vi "Costruisci rampa.vi"(11 "Cluster rampa":T2={"Numero step totali"=10.0, "Tempo step [s]"=1.0, "Freno"={"MARCIA"=FALSE, "Control Type"=enum."Speed [RPM]", "RIF iniziale %"=100.0, "RIF finale %"=100.0}, "ALIMENTATORE 1"={"MARCIA"=FALSE, "RIF V iniziale"=100.0, "RIF V FINALE"=100.0, "RIF F INIZIALE"=100.0, "RIF F finale"=100.0}, "ALIMENTATORE 2"={"MARCIA"=FALSE, "RIF V iniziale"=0.0, "RIF F iniziale"=0.0, "RIF V finale"=0.0, "RIF F finale"=0.0}, "Tipo prova"="[2] A CARICO", "Caratteristiche step"={"Attendi stabilizz."=TRUE, "Acq. fine step?"=TRUE, "Acq. automatiche"=FALSE, "PID FRENO"=TRUE, "PID ALIMENTATORE 1"=TRUE, "PID ALIMENTATORE 2"=FALSE, "CAMBIA PROVA SE EQ. TERMICO"=FALSE}}) -> (3 "Array":string[][](array[string]))   [LabVIEW 2019]
uses:
  controls/STEP.ctl
  controls/Caratteristiche step.ctl
  <vilib>/gmath/NI_Gmath.lvlib
panel:
  in  "NUOVO STEP":T3 {"Tempo Step[s]" format="%#.1f"}
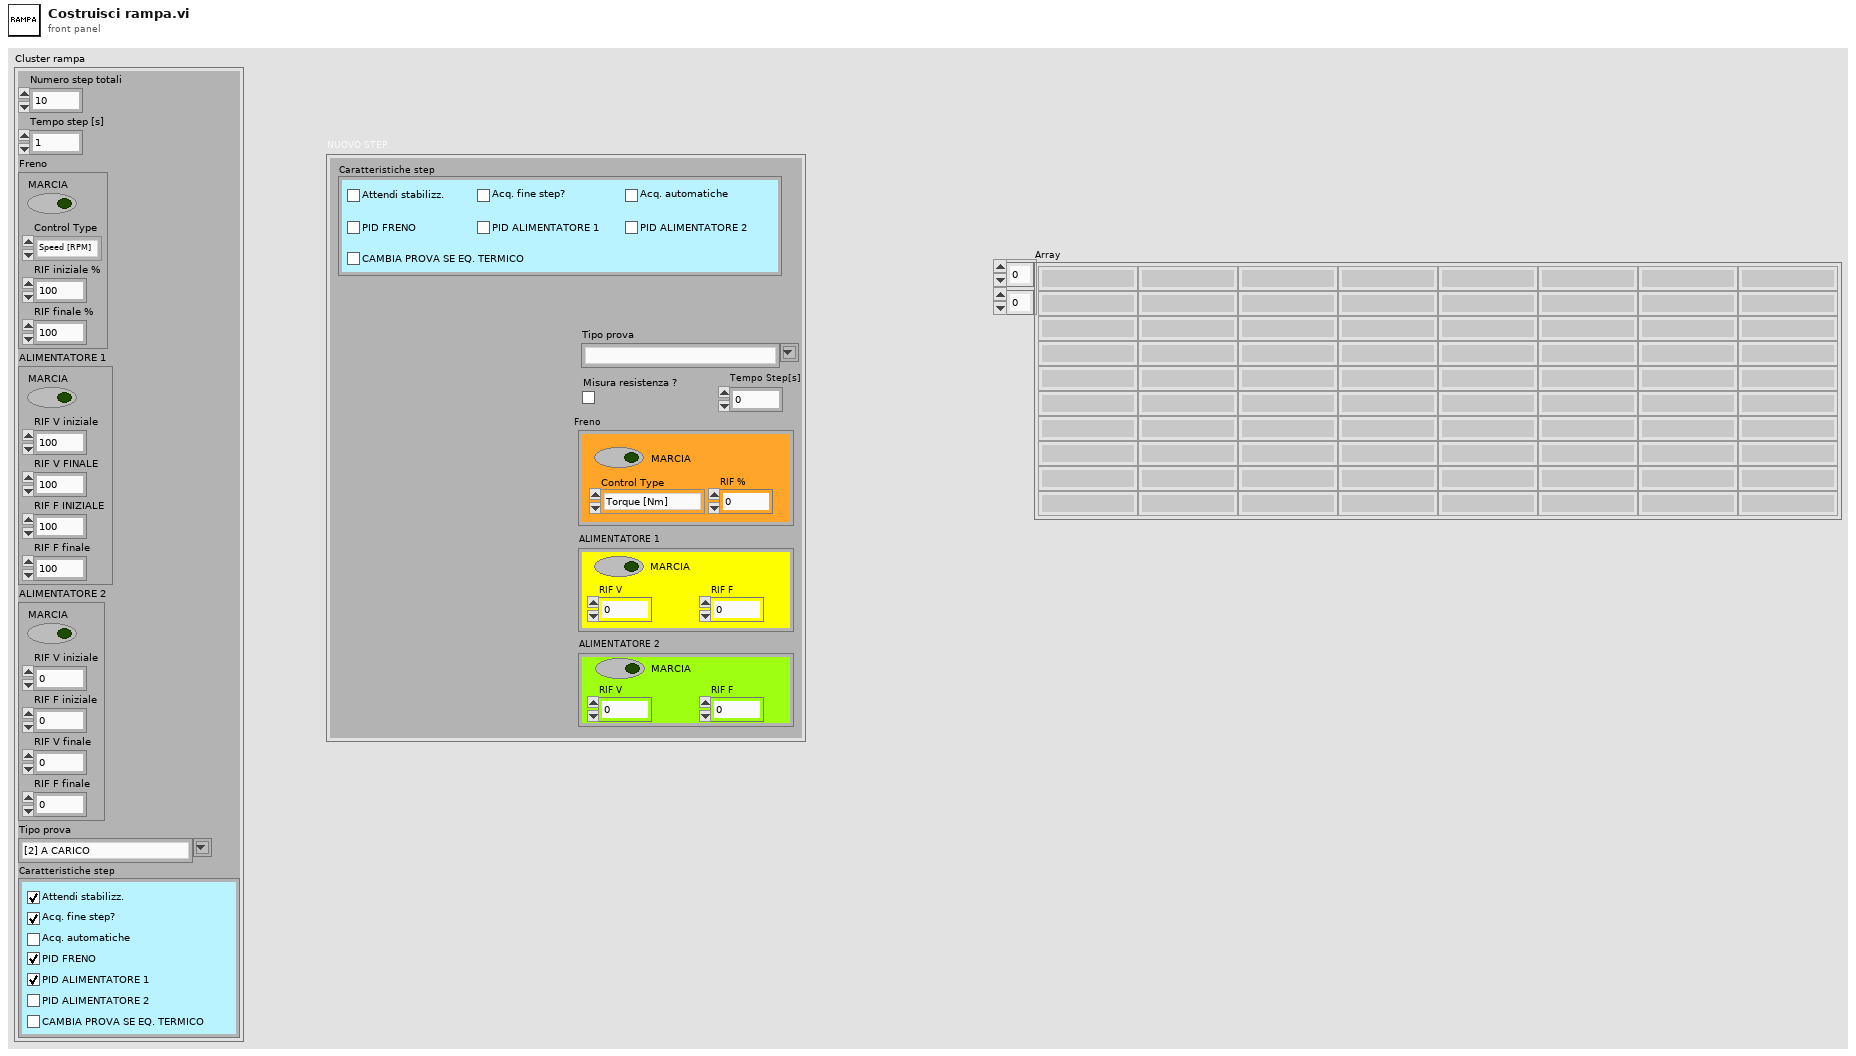
[diagram p1: front panel]
types:
  T1 = typedef "Caratteristiche step.ctl" = cluster{"Attendi stabilizz.":bool, "Acq. fine step?":bool, "Acq. automatiche":bool, "PID FRENO":bool, "PID ALIMENTATORE 1":bool, "PID ALIMENTATORE 2":bool, "CAMBIA PROVA SE EQ. TERMICO":bool}
  T2 = cluster{"Numero step totali":dbl, "Tempo step [s]":dbl, "Freno":cluster{"MARCIA":bool, "Control Type":enum32{"Torque [Nm]", "Power [W]", "Speed [RPM]", "Corrente [A]"}, "RIF iniziale %":dbl, "RIF finale %":dbl}, "ALIMENTATORE 1":cluster{"MARCIA":bool, "RIF V iniziale":dbl, "RIF V FINALE":dbl, "RIF F INIZIALE":dbl, "RIF F finale":dbl}, "ALIMENTATORE 2":cluster{"MARCIA":bool, "RIF V iniziale":dbl, "RIF F iniziale":dbl, "RIF V finale":dbl, "RIF F finale":dbl}, "Tipo prova":string, "Caratteristiche step":T1}
  T3 = typedef "STEP.ctl" = cluster{"Tipo prova":string, "Misura resistenza ?":bool, "Tempo Step[s]":dbl, "Freno":cluster{"MARCIA":bool, "Control Type":enum32{"Torque [Nm]", "Power [W]", "Speed [RPM]", "Corrente [A]"}, "RIF %":dbl}, "ALIMENTATORE 1":cluster{"MARCIA":bool, "RIF V":dbl, "RIF F":dbl}, "ALIMENTATORE 2":cluster{"MARCIA":bool, "RIF V":dbl, "RIF F":dbl}, "Caratteristiche step":T1}
  T4 = cluster{"MARCIA":bool, "Control Type":enum32{"Torque [Nm]", "Power [W]", "Speed [RPM]", "Corrente [A]"}, "RIF iniziale %":dbl, "RIF finale %":dbl}
  T5 = cluster{"MARCIA":bool, "RIF V iniziale":dbl, "RIF V FINALE":dbl, "RIF F INIZIALE":dbl, "RIF F finale":dbl}
  T6 = cluster{"MARCIA":bool, "RIF V iniziale":dbl, "RIF F iniziale":dbl, "RIF V finale":dbl, "RIF F finale":dbl}
  T7 = enum32{"Torque [Nm]", "Power [W]", "Speed [RPM]", "Corrente [A]"}
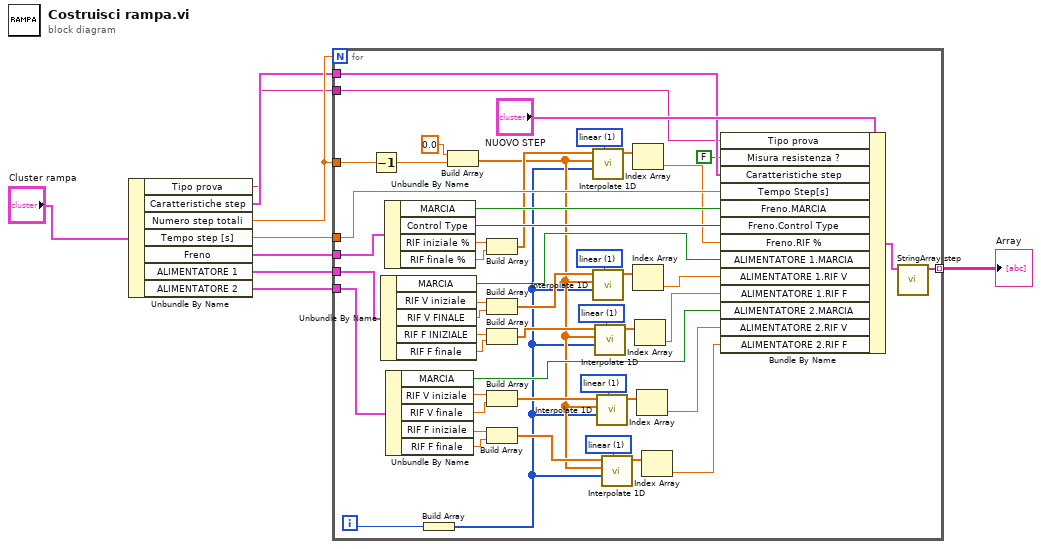
[diagram p0: block diagram]
diagram:
  n1 = Unbundle By Name("Cluster rampa") -> ("Tipo prova"=w1:string, "Caratteristiche step"=w2:T1, "Numero step totali"=w4:dbl, "Tempo step [s]"=w6:dbl, "Freno"=w9:T4, "ALIMENTATORE 1"=w8:T5, "ALIMENTATORE 2"=w7:T6)
  n2 = for {
    N: w4 -> [_]
    tunnel: w9 -> [w59]
    tunnel: w8 -> [w58]
    tunnel: w7 -> [w57]
    tunnel: w6 -> [w51]
    tunnel: [w52] -> w5 mode=indexing
    tunnel: w4 -> [w46]
    tunnel: w2 -> [w12]
    tunnel: w1 -> [w10]
    i -> [w45]
    w19 = 1 items=["nearest", "linear", "spline", "cubic Hermite", "Lagrange"] ("method")
    w23 = 1 items=["nearest", "linear", "spline", "cubic Hermite", "Lagrange"] ("method")
    w28 = 1 items=["nearest", "linear", "spline", "cubic Hermite", "Lagrange"] ("method")
    w32 = 1 items=["nearest", "linear", "spline", "cubic Hermite", "Lagrange"] ("method")
    w44 = 1 items=["nearest", "linear", "spline", "cubic Hermite", "Lagrange"] ("method")
    n3 = Decrement(x=w46) -> (x-1=w13:dbl)
    n4 = Unbundle By Name(w58) -> ("MARCIA"=w31:bool, "RIF V iniziale"=w41:dbl, "RIF V FINALE"=w40:dbl, "RIF F INIZIALE"=w39:dbl, "RIF F finale"=w38:dbl)
    n5 = Unbundle By Name(w59) -> ("MARCIA"=w55:bool, "Control Type"=w54:T7, "RIF iniziale %"=w50:dbl, "RIF finale %"=w49:dbl)
    n6 = Unbundle By Name(w57) -> ("MARCIA"=w22:bool, "RIF V iniziale"=w37:dbl, "RIF V finale"=w36:dbl, "RIF F iniziale"=w35:dbl, "RIF F finale"=w34:dbl)
    n7 = Build Array(w45) -> (w15:i32[])
    n8 = Build Array(0.0 ("element"), w13) -> (w16:dbl[])
    n9 = Build Array(w50, w49) -> (w48:dbl[])
    n10 = Build Array(w41, w40) -> (w30:dbl[])
    n11 = Build Array(w39, w38) -> (w26:dbl[])
    n12 = Build Array(w37, w36) -> (w21:dbl[])
    n13 = Build Array(w35, w34) -> (w17:dbl[])
    n14 = call <vilib>:"Interpolate 1D.vi"("method"=w44, "xi"=w15, "X"=w16, "Y"=w48) -> ("yi"=w43:dbl[])  [unwired: 5 in, 2 out]
    n15 = call <vilib>:"Interpolate 1D.vi"("method"=w32, "xi"=w15, "X"=w16, "Y"=w30) -> ("yi"=w33:dbl[])  [unwired: 5 in, 2 out]
    n16 = call <vilib>:"Interpolate 1D.vi"("method"=w28, "xi"=w15, "X"=w16, "Y"=w26) -> ("yi"=w27:dbl[])  [unwired: 5 in, 2 out]
    n17 = call <vilib>:"Interpolate 1D.vi"("method"=w23, "xi"=w15, "X"=w16, "Y"=w21) -> ("yi"=w24:dbl[])  [unwired: 5 in, 2 out]
    n18 = call <vilib>:"Interpolate 1D.vi"("method"=w19, "xi"=w15, "X"=w16, "Y"=w17) -> ("yi"=w18:dbl[])  [unwired: 5 in, 2 out]
    n19 = Index Array(array=w43) -> (element=w42:dbl)  [unwired: 1 in]
    n20 = Index Array(array=w33) -> (element=w29:dbl)  [unwired: 1 in]
    n21 = Index Array(array=w27) -> (element=w25:dbl)  [unwired: 1 in]
    n22 = Index Array(array=w24) -> (element=w20:dbl)  [unwired: 1 in]
    n23 = Index Array(array=w18) -> (element=w14:dbl)  [unwired: 1 in]
    n24 = Bundle By Name(cluster="NUOVO STEP", "Tipo prova"=w10, "Misura resistenza ?"=FALSE, "Caratteristiche step"=w12, "Tempo Step[s]"=w51, "Freno.MARCIA"=w55, "Freno.Control Type"=w54, "Freno.RIF %"=w42, "ALIMENTATORE 1.MARCIA"=w31, "ALIMENTATORE 1.RIF V"=w29, "ALIMENTATORE 1.RIF F"=w25, "ALIMENTATORE 2.MARCIA"=w22, "ALIMENTATORE 2.RIF V"=w20, "ALIMENTATORE 2.RIF F"=w14) -> (w53:T3)
    n25 = call "StringArray step.vi"("NUOVO STEP"=w53) -> ("Array"=w52:string[])  [unwired: 10 in]
  }
  "Array" <- w5
